vi "ServerReflection ServerReflectionInfo Write.vi"(8 "error in":errorcluster, 10 "Request Data":T1, 11 "Call ID in":T2) -> (0 "error out":errorcluster, 2 "Success":bool, 3 "Call ID":T2)   [LabVIEW 2025, in "reflection_client.lvlib"]
uses:
  reflection_client.lvlib
  <vilib>/gRPC/LabVIEW gRPC Library/Shared/grpcId.ctl
  RPC Messages/grpc_reflection_v1alpha_ServerReflectionRequest.ctl
  RPC Messages/grpc_reflection_v1alpha_ServerReflectionRequest_message_request/grpc_reflection_v1alpha_ServerReflectionRequest_message_request.lvclass
  RPC Messages/grpc_reflection_v1alpha_ServerReflectionRequest_message_request/grpc_reflection_v1alpha_ServerReflectionRequest_message_request.lvclass/grpc_reflection_v1alpha_ServerReflectionRequest_message_request.ctl
  9647bdd3-bda2-4565-bbb9-d670be58a455.vi
  RPC Messages/grpc_reflection_v1alpha_ServerReflectionRequest_message_request/GetActiveFieldIndex.vi
  RPC Messages/grpc_reflection_v1alpha_ServerReflectionRequest_message_request/Getfile_by_filename.vi
  RPC Messages/grpc_reflection_v1alpha_ServerReflectionRequest_message_request/Getfile_containing_symbol.vi
  RPC Messages/grpc_reflection_v1alpha_ServerReflectionRequest_message_request/Getfile_containing_extension.vi
  RPC Messages/RichToFlatgrpc_reflection_v1alpha_ExtensionRequest.vi
  RPC Messages/grpc_reflection_v1alpha_ServerReflectionRequest_message_request/Getall_extension_numbers_of_type.vi
  RPC Messages/grpc_reflection_v1alpha_ServerReflectionRequest_message_request/Getlist_services.vi
  <vilib>/gRPC/LabVIEW gRPC Library/Shared/TranslateGrpcError.vi
  <vilib>/gRPC/LabVIEW gRPC Library/Server API/Server/Get Server DLL Path.vi
  <vilib>/Utility/error.llb/Error Cluster From Error Code.vi
  <vilib>/gRPC/LabVIEW gRPC Library/grpc-lvsupport-release.lvlib
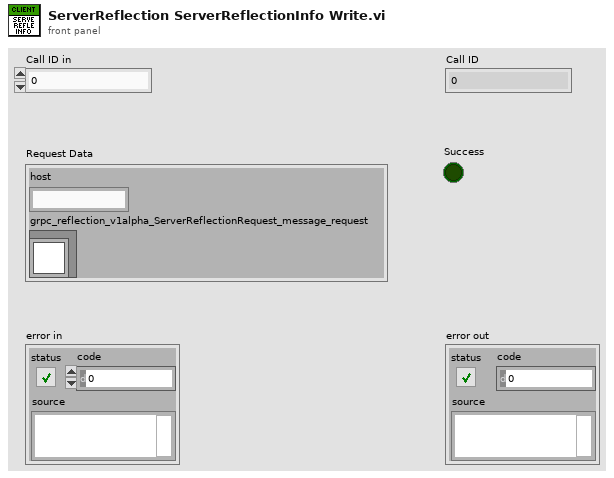
[diagram p1: front panel]
types:
  T1 = typedef "reflection_client.lvlib/grpc_reflection_v1alpha_ServerReflectionRequest.ctl" = cluster{"host":string, "grpc_reflection_v1alpha_ServerReflectionRequest_message_request":refnum<class "grpc_reflection_v1alpha_ServerReflectionRequest_message_request.lvclass">}
  T2 = typedef "grpc-lvsupport-release.lvlib/grpcId.ctl" = u64
  T3 = typedef "reflection_client.lvlib/grpc_reflection_v1alpha_ServerReflectionRequest_Flat.ctl" = cluster{"host":string, "grpc_reflection_v1alpha_ServerReflectionRequest_message_request_selected_index":i32, "file_by_filename":string, "file_containing_symbol":string, "file_containing_extension":T4, "all_extension_numbers_of_type":string, "list_services":string}
  T4 = typedef "reflection_client.lvlib/grpc_reflection_v1alpha_ExtensionRequest_Flat.ctl" = cluster{"containing_type":string, "extension_number":i32}
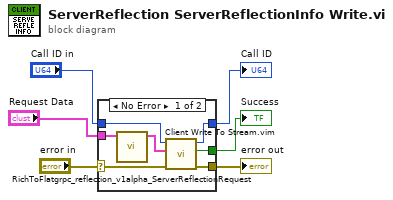
[diagram p0: block diagram]
diagram:
  n1 = case shown="No Error" "error in" {
    selector: "error in" -> [w13 w14]
    tunnel: [w12 w14] -> w5
    tunnel: "Call ID in" -> [w11 w15]
    tunnel: [w10 w15] -> w3
    tunnel: "Request Data" -> [w8 _]
    tunnel: [w9 _] -> w1
    frame No Error {
      n2 = call "RichToFlatgrpc_reflection_v1alpha_ServerReflectionRequest.vi"("InputCluster"=w8) -> ("OutputCluster"=w7:T3)  [unwired: 10 in]
      n3 = call "Client Write To Stream.vim"("error in"=w13, "Request Data"=w7, "Call ID in"=w11) -> ("error out"=w12:errorcluster, "Success"=w9:bool, "Call ID out"=w10:u64)  [unwired: 6 in]
    }
    frame Error {
    }
  }
  "error out" <- w5
  "Call ID" <- w3
  "Success" <- w1
